vi "SeleteUUT_DataSave2.vi"(8 "error in (no error)":errorcluster caption="错误输入（无错误）", 10 "选择测试板数据":dbl, 11 "real report 3":refnum<vi>) -> (0 "error out":errorcluster caption="错误输出", 2 "项名":string[][](array[string]), 3 "引用输出":refnum<vi>)   [LabVIEW 2018]
panel:
  out "大小":i32[](array[numeric])
  out "元素":i32
  out "步骤":i32
  out "数组":i32[](array[numeric])
  in  "real report 2":i32(listbox) caption="real report"
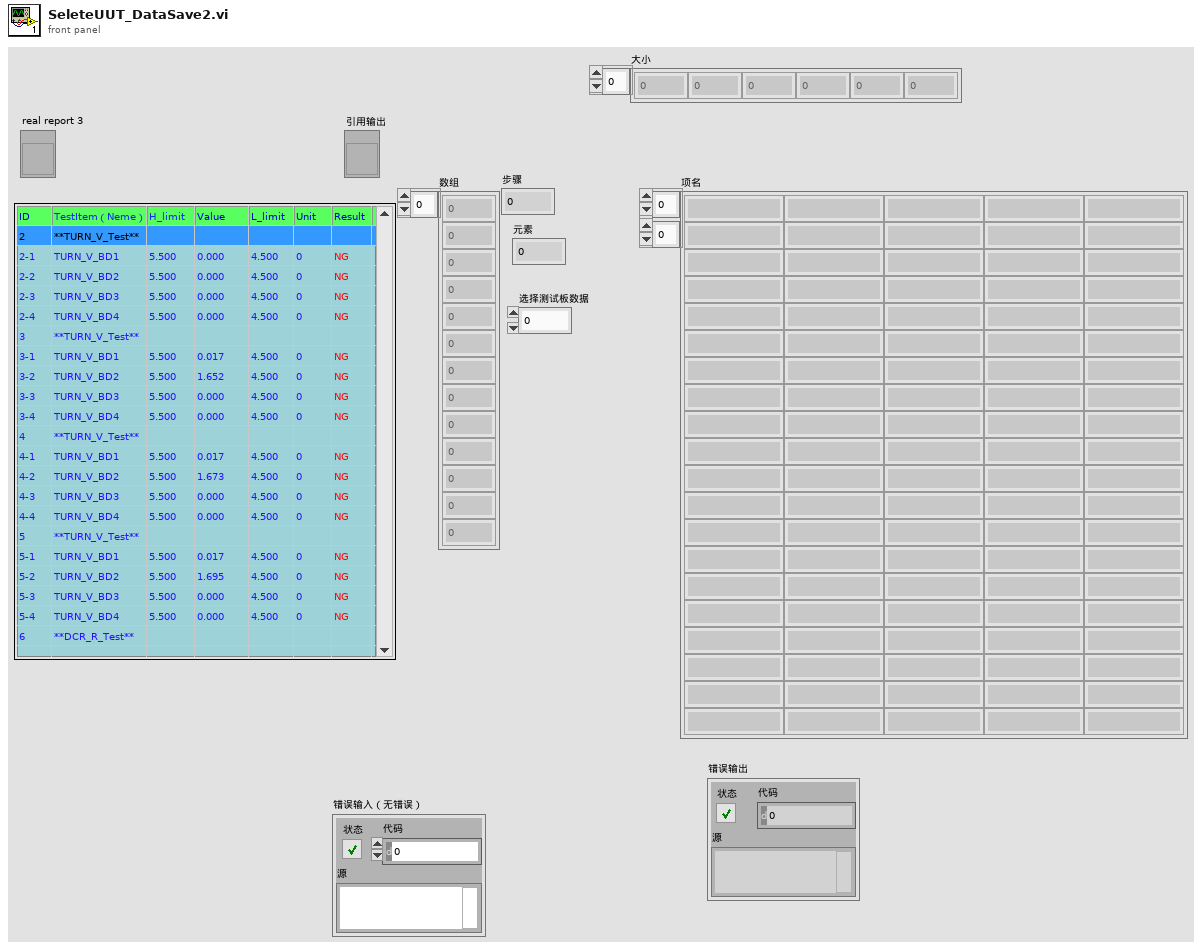
[diagram p1: front panel]
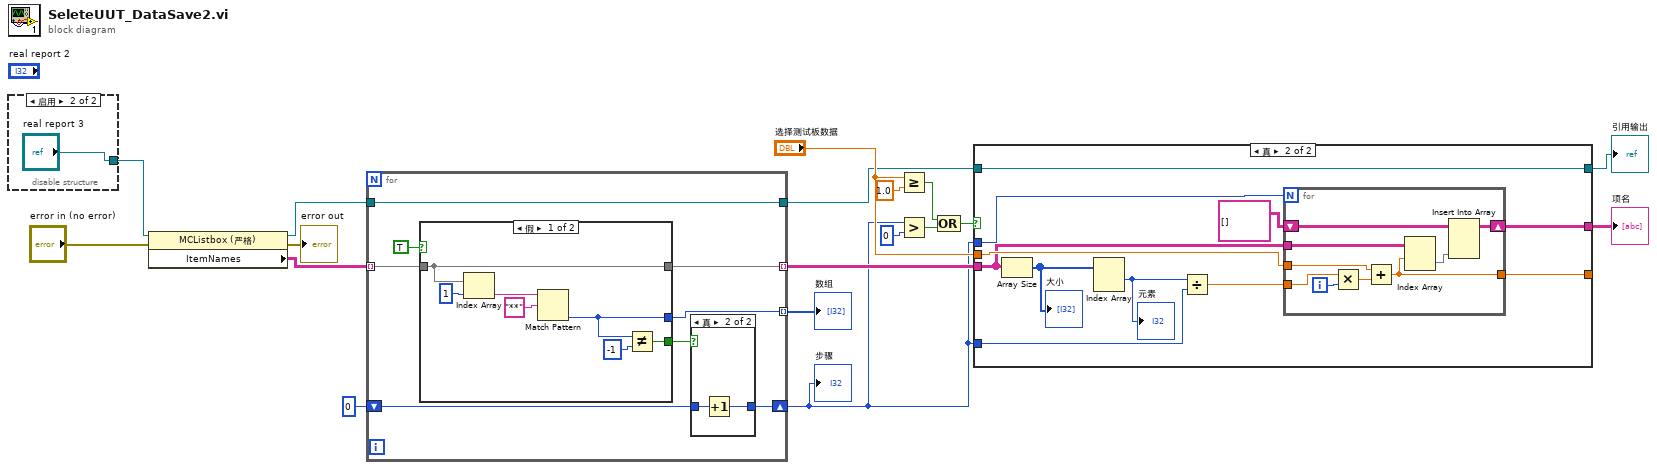
[diagram p0: block diagram]
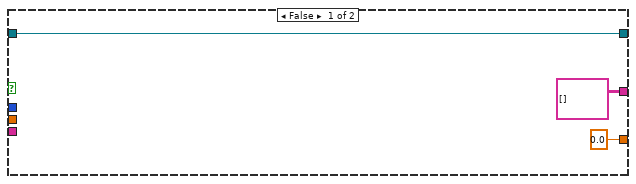
[diagram p2: hidden frame]
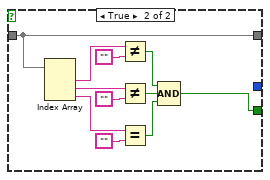
[diagram p3: hidden frame]
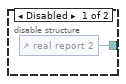
[diagram p5: hidden frame]
diagram:
  n1 = disable-structure shown="启用" {
    disable-tunnel: [w19 "real report 3"] -> w18
    frame Disabled {
      n2 = control-ref of="real report 2"() -> (w19:refnum<vi>)
    }
    frame Enabled {
    }
  }
  n3 = property class="MCListbox (严格)"(reference=w18, error in="error in (no error)") -> (reference out=w6:refnum<vi>, error out=→"error out":errorcluster, "ItemNames"=w13:string[][])
  n4 = for {
    tunnel: w13 -> [w25] mode=indexing
    tunnel: [w24] -> w12 mode=indexing
    shift-right: [w27] -> w3
    shift-left: 0 -> [w28]
    tunnel: [w22] -> w9 mode=indexing
    tunnel: [w26] -> w5
    tunnel: w6 -> [w26]
    n5 = case shown="假" TRUE {
      tunnel: [w29 w36] -> w22
      tunnel: [w32 w41] -> w21
      tunnel: w25 -> [w29 w36]
      tunnel: [w30 _] -> w24
      frame False {
        n6 = Index Array(array=w29, index=1 ("索引")) -> (element=w31:string)
        n7 = Match Pattern(string=w31, regular expression="**" ("正则表达式")) -> (offset past match=w30:i32)  [unwired: 1 in, 3 out]
        n8 = Not Equal?(x=w30, y=-1) -> (x != y?=w32:bool)
      }
      frame True {
        n9 = Index Array(array=w36) -> (element #1=w46:string, element #2=w44:string, element #3=w38:string)  [unwired: 3 in]
        n10 = Not Equal?(x=w46, y="") -> (x != y?=w43:bool)
        n11 = Not Equal?(x=w44, y="") -> (x != y?=w42:bool)
        n12 = Equal?(x=w38, y="") -> (x = y?=w37:bool)
        n13 = Compound Arithmetic op=AND ("复合运算")(w43, w42, w37) -> (w41:bool)
      }
    }
    n14 = case shown="真" w21 {
      tunnel: w28 -> [w47 w49]
      tunnel: [w47 w48] -> w27
      frame False {
      }
      frame True {
        n15 = Increment(x=w49) -> (x+1=w48:i32)
      }
    }
  }
  "数组" <- w12
  "步骤" <- w3
  n16 = Greater Or Equal?(x="选择测试板数据", y=1.0) -> (x >= y?=w17:bool)
  n17 = Greater?(x=w3, y=0) -> (0:w15:bool)
  n18 = Compound Arithmetic op=OR ("复合运算")(w17, w15) -> (w10:bool)
  n19 = case shown="真" w10 {
    tunnel: [string[][] [] ("项名") w60] -> w4
    tunnel: w3 -> [_ w59]
    tunnel: "选择测试板数据" -> [_ w57]
    tunnel: [0.0 w56] -> _
    tunnel: w9 -> [_ w55]
    tunnel: [w50 w54] -> w7
    tunnel: w5 -> [w50 w54]
    tunnel: w3 -> [_ w53]
    frame False {
    }
    frame True {
      n20 = Array Size(array=w55) -> (size(s)=w63:i32[])
      "大小" <- w63
      n21 = Index Array(array=w63) -> (element #1=w62:i32)  [unwired: 2 in, 1 out]
      "元素" <- w62
      n22 = Divide(x=w62, y=w59) -> (x/y=w58:dbl)
      n23 = for {
        N: w53 -> [_]
        tunnel: w55 -> [w72]
        tunnel: w58 -> [w71]
        shift-right: [w70] -> w60
        shift-left: string[][] [] ("项名") -> [w69]
        tunnel: w57 -> [w66]
        tunnel: [w64] -> w56
        i -> [w67]
        n24 = Multiply(x=w71, y=w67) -> (x*y=w65:dbl)
        n25 = Add(x=w66, y=w65) -> (x+y=w64:dbl)
        n26 = Index Array(array=w72, index (row)=w64) -> (element=w68:string[])  [unwired: 1 in]
        n27 = Insert Into Array(array=w69, new element=w68) -> (w70:string[][])  [unwired: 2 in]
      }
    }
  }
  "引用输出" <- w7
  "项名" <- w4
